vi "MultiJoint по линии.vi"() -> ()   [LabVIEW 2020]
panel:
  in  "Shoulder Size 3":dbl
  in  "Shoulder Size 2":dbl
  in  "1 joint 2":dbl(slide) scale=0.0..180.0
  in  "Shoulder Size":dbl
  in  "4 joint":dbl(slide) scale=0.0..180.0
  in  "3 joint":dbl(slide) scale=0.0..180.0
  in  "2 joint":dbl(slide) scale=0.0..180.0
  in  "1 joint":dbl(slide) scale=0.0..180.0
  out "XY Graph":cluster{dbl[], dbl[]}(graph)
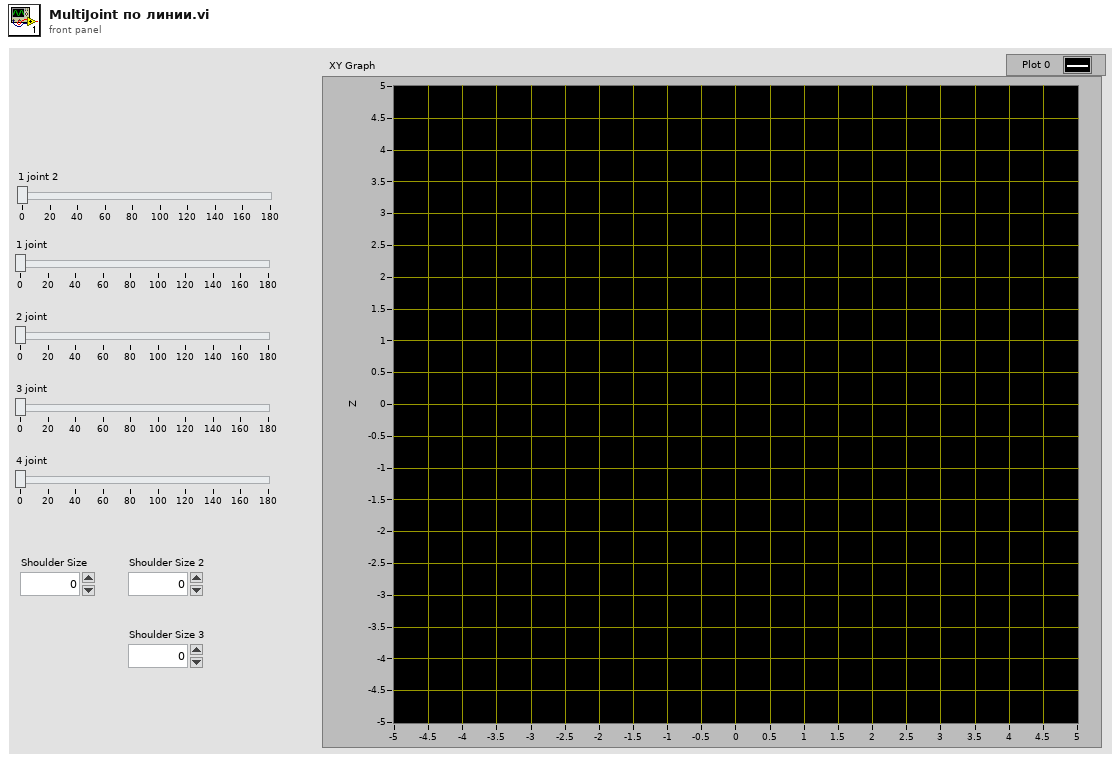
[diagram p1: front panel]
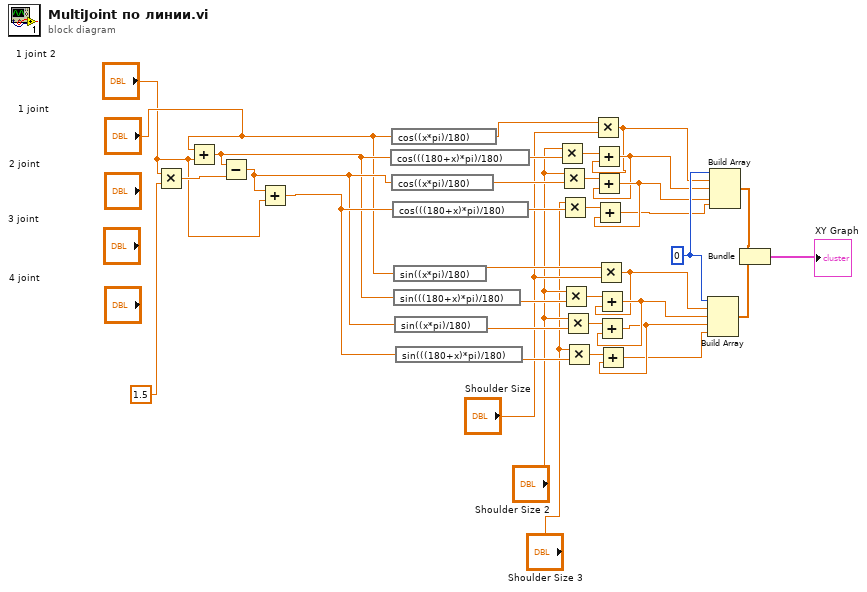
[diagram p0: block diagram]
diagram:
  w31 = 0
  n1 = Multiply(x="1 joint 2", y=1.5) -> (x*y=w3:dbl)
  n2 = Add(x="1 joint", y="1 joint 2") -> (x+y=w22:dbl)
  n3 = Subtract(x=w22, y=w3) -> (x-y=w23:dbl)
  n4 = Add(x=w23, y="1 joint 2") -> (x+y=w24:dbl)
  n5 = expression code="cos(((180+x)*pi)/180)"(w22) -> (w18:dbl)
  n6 = expression code="cos((x*pi)/180)"("1 joint") -> (w33:dbl)
  n7 = expression code="cos((x*pi)/180)"(w23) -> (w13:dbl)
  n8 = expression code="cos(((180+x)*pi)/180)"(w24) -> (w14:dbl)
  n9 = expression code="sin((x*pi)/180)"("1 joint") -> (w32:dbl)
  n10 = expression code="sin(((180+x)*pi)/180)"(w22) -> (w16:dbl)
  n11 = expression code="sin((x*pi)/180)"(w23) -> (w9:dbl)
  n12 = expression code="sin(((180+x)*pi)/180)"(w24) -> (w8:dbl)
  n13 = Multiply(x="Shoulder Size 2", y=w18) -> (x*y=w19:dbl)
  n14 = Multiply(x="Shoulder Size 2", y=w13) -> (x*y=w15:dbl)
  n15 = Multiply(x="Shoulder Size 3", y=w14) -> (x*y=w12:dbl)
  n16 = Multiply(x="Shoulder Size 2", y=w16) -> (x*y=w17:dbl)
  n17 = Multiply(x="Shoulder Size 2", y=w9) -> (x*y=w10:dbl)
  n18 = Multiply(x="Shoulder Size 3", y=w8) -> (x*y=w11:dbl)
  n19 = Multiply(x=w33, y="Shoulder Size") -> (x*y=w21:dbl)
  n20 = Add(x=w19, y=w21) -> (x+y=w29:dbl)
  n21 = Add(x=w15, y=w29) -> (x+y=w30:dbl)
  n22 = Add(x=w12, y=w30) -> (x+y=w28:dbl)
  n23 = Multiply(x=w32, y="Shoulder Size") -> (x*y=w20:dbl)
  n24 = Add(x=w17, y=w20) -> (x+y=w27:dbl)
  n25 = Add(x=w10, y=w27) -> (x+y=w26:dbl)
  n26 = Add(x=w11, y=w26) -> (x+y=w25:dbl)
  n27 = Build Array(w31, w20, w27, w26, w25) -> (w34:dbl[])
  n28 = Build Array(w31, w21, w29, w30, w28) -> (w35:dbl[])
  n29 = Bundle(w35, w34) -> (→"XY Graph":cluster{dbl[], dbl[]})  [unwired: 1 in]
